vi "Wait Async Do.vi"(8 "error in (no error)":errorcluster, 9 "Async Message":refnum<class "Async Message.lvclass">, 10 "VI Refnum":refnum<vi>, 11 "Async Methods Actor in":refnum<class "Async Methods Actor.lvclass">) -> (0 "error out":errorcluster, 3 "Async Methods Actor out":refnum<class "Async Methods Actor.lvclass">)   [LabVIEW 2023, in "Async Methods Actor.lvlib" / "Async Methods Actor.lvclass"]
uses:
  Async Methods Actor.lvclass
  <vilib>/ActorFramework/Actor/Actor.lvclass
  Async Methods Actor Messages/Async Message/Async Message.lvclass
  C:/Program Files/National Instruments/LabVIEW 2023/vi.lib/ActorFramework/Actor/Actor.lvclass
  <vilib>/ActorFramework/Actor/Actor.lvclass/Actor.ctl
  <vilib>/ActorFramework/Message Enqueuer/Message Enqueuer.lvclass/Message Enqueuer.ctl
  Async Methods Actor Messages/Async Message/Async Message.lvclass/Async Message.ctl
  Async Methods Actor Messages/Completion Notification Msg/Completion Notification Msg.lvclass/Completion Notification Msg.ctl
  <vilib>/ActorFramework/Report Error Msg/Report Error Msg.lvclass/Report Error Msg.ctl
  Async Methods Actor Messages/Remove Async Message from Map Msg/Remove Async Message from Map Msg.lvclass/Remove Async Message from Map Msg.ctl
  Async Methods Actor Messages/Acknowledge Completion Msg/Acknowledge Completion Msg.lvclass/Acknowledge Completion Msg.ctl
  Async Methods Actor Messages/Async Message/Read Report Errors.vi
  Async Methods Actor Messages/Async Message/Read Notify Completion.vi
  Async Methods Actor Messages/Async Message/Write Async Method Error.vi
  <vilib>/ActorFramework/Message Enqueuer/Init from Existing Queue.vi
  <vilib>/ActorFramework/Message Enqueuer/Enqueue.vi
  <vilib>/ActorFramework/Message Enqueuer/Equals Not A Refnum.vi
  Async Methods Actor Messages/Completion Notification Msg/Write Async Method Error.vi
  <vilib>/ActorFramework/Report Error Msg/Report Error Msg.lvclass
  C:/Program Files/National Instruments/LabVIEW 2023/vi.lib/ActorFramework/Message/Message.lvclass
  Async Methods Actor Messages/Remove Async Message from Map Msg/Remove Async Message from Map Msg.lvclass
  Async Methods Actor Messages/Acknowledge Completion Msg/Acknowledge Completion Msg.lvclass
  <vilib>/Utility/LVClass/Get LV Class Name.vi
  <resource>/AFDebug/Generate Trace for Message.vi
  <vilib>/ActorFramework/Message Priority Queue/Priority Enqueue.vi
  <vilib>/ActorFramework/Message Enqueuer/Message Enqueuer.lvclass
  Async Methods Actor Messages/Notify Completion Msg/Notify Completion Msg.lvclass
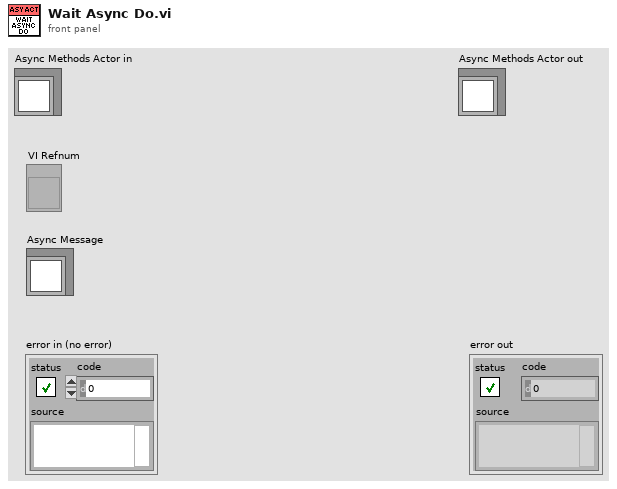
[diagram p1: front panel]
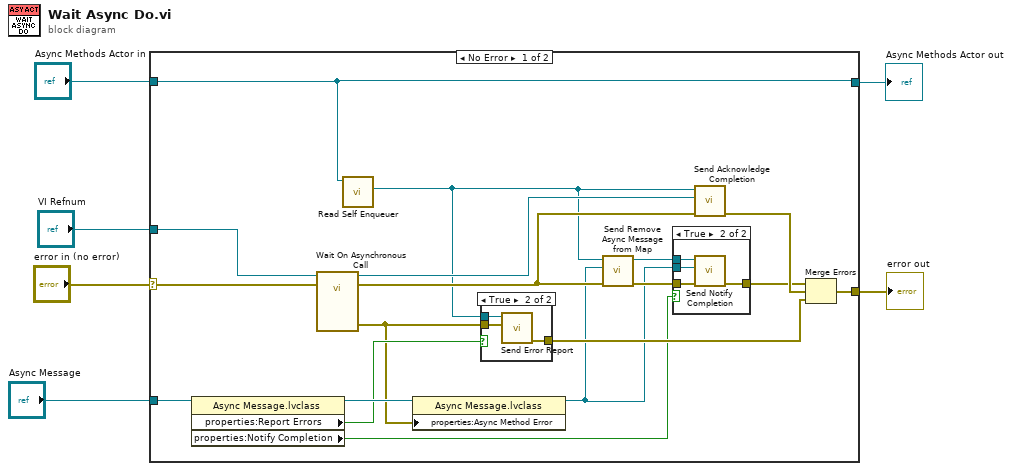
[diagram p0: block diagram]
diagram:
  n1 = case shown="No Error" "error in (no error)" {
    selector: "error in (no error)" -> [w24 w34]
    tunnel: "VI Refnum" -> [w23 _]
    tunnel: [w22 w34] -> w4
    tunnel: "Async Methods Actor in" -> [w18 w33]
    tunnel: [w18 w33] -> w2
    tunnel: "Async Message" -> [w17 _]
    frame No Error {
      n2 = property class="Async Message.lvclass"(reference=w17) -> (reference out=w13:refnum<class "Async Message.lvclass">, "properties:Report Errors"=w9:bool, "properties:Notify Completion"=w10:bool)  [unwired: 1 in, 1 out]
      n3 = call-by-ref "Wait On Asynchronous Call"(reference=w23, error in=w24) -> (reference out=w21:refnum<vi>, error out=w19:errorcluster, 0:"error out"=w7:errorcluster)  [unwired: 10 in, 1 out]
      n4 = call <vilib>:"Read Self Enqueuer.vi"("Actor"=w18) -> ("Self Enqueuer"=w12:refnum<class "Message Enqueuer.lvclass">)  [unwired: 10 in]
      n5 = property class="Async Message.lvclass"(reference=w13, "properties:Async Method Error"=w7) -> (reference out=w8:refnum<class "Async Message.lvclass">)  [unwired: 1 in, 1 out]
      n6 = case shown="True" w9 {
        tunnel: w7 -> [_ w27]
        tunnel: w12 -> [_ w26]
        tunnel: [_ w25] -> w11
        frame False {
        }
        frame True {
          n7 = call <vilib>:"Send Error Report.vi"("Error From Sender"=w27, "Message Enqueuer"=w26) -> ("error out"=w25:errorcluster)  [unwired: 9 in]
        }
      }
      n8 = call "Send Remove Async Message from Map.vi"("error in (no error)"=w19, "Message"=w8, "Message Enqueuer in"=w12) -> ("error out"=w16:errorcluster, "Message Enqueuer out"=w14:refnum<class "Message Enqueuer.lvclass">)  [unwired: 7 in]
      n9 = case shown="True" w10 {
        tunnel: w16 -> [w28 w32]
        tunnel: [w28 w31] -> w15
        tunnel: w14 -> [_ w30]
        tunnel: w8 -> [_ w29]
        frame False {
        }
        frame True {
          n10 = call "Send Notify Completion.vi"("error in (no error)"=w32, "Async Message"=w29, "Message Enqueuer in"=w30) -> ("error out"=w31:errorcluster)  [unwired: 7 in, 1 out]
        }
      }
      n11 = call "Send Acknowledge Completion.vi"("error in (no error)"=w19, "VI Refnum"=w21, "Message Enqueuer in"=w12) -> ("error out"=w20:errorcluster)  [unwired: 7 in, 1 out]
      n12 = Merge Errors(w15, w20, w11) -> (w22:errorcluster)
    }
    frame Error {
    }
  }
  "error out" <- w4
  "Async Methods Actor out" <- w2
